vi "drive_setOut.vi"(11 "Drive_Outputs":T1) -> ()   [LabVIEW 2013]
uses:
  drive_outputs.ctl
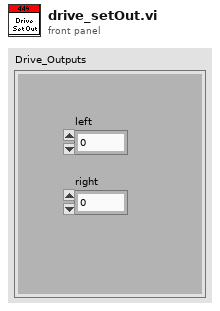
[diagram p1: front panel]
types:
  T1 = typedef "drive_outputs.ctl" = cluster{"left":dbl, "right":dbl}
  T2 = typedef "WPI_MotorControlDeviceRef.ctl" = cluster{"DeviceStatus":errorcluster, "Type":enum16{"PWM", "CAN"}, "PWM":cluster{"Digital Module":T3, "PWM Channel":T4, "DeadBand":T5}, "CAN":cluster{"Device Number":u8, "Control Mode":T6, "Semaphore":T7, "Max Vout":dbl}, "Invert":bool, "TransformRef":T8, "InvTransformRef":T8}
  T3 = typedef "FPGA_TypedefDigitalModule.ctl" = enum16{"Digital Module 1", "Digital Module 2"}
  T4 = typedef "FPGA_DIOPWMChannel.ctl" = enum8{"PWM 1", "PWM 2", "PWM 3", "PWM 4", "PWM 5", "PWM 6", "PWM 7", "PWM 8", "PWM 9", "PWM 10", "Invalid"}
  T5 = typedef "WPI_PWMDeadband.ctl" = cluster{"Name":string, "maxPositivePwm":i32, "minPositivePwm":i32, "centerPwm":i32, "maxNegativePwm":i32, "minNegativePwm":i32, "angularRange":u16}
  T6 = typedef "WPI_CANJaguar_ControlMode.ctl" = enum8{"Percent VBus", "Current", "Speed", "Position", "Voltage"}
  T7 = typedef "Semaphore RefNum" = refnum<k1>
  T8 = typedef "WPI_PWMTransform_ConPane.ctl" = refnum<vi>
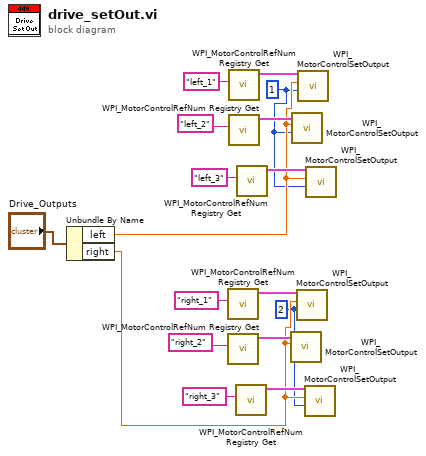
[diagram p0: block diagram]
diagram:
  w1 = u8 2 ("Sync Group")
  w2 = u8 1 ("Sync Group")
  n1 = Unbundle By Name("Drive_Outputs") -> ("left"=w10:dbl, "right"=w3:dbl)
  n2 = call <vilib>:"WPI_MotorControlRefNum Registry Get.vi"("refnum name"="right_1") -> ("MotorControlDevRef"=w9:T2)  [unwired: 9 in, 1 out]
  n3 = call <vilib>:"WPI_MotorControlRefNum Registry Get.vi"("refnum name"="right_2") -> ("MotorControlDevRef"=w7:T2)  [unwired: 9 in, 1 out]
  n4 = call <vilib>:"WPI_MotorControlRefNum Registry Get.vi"("refnum name"="left_1") -> ("MotorControlDevRef"=w16:T2)  [unwired: 9 in, 1 out]
  n5 = call <vilib>:"WPI_MotorControlRefNum Registry Get.vi"("refnum name"="left_2") -> ("MotorControlDevRef"=w14:T2)  [unwired: 9 in, 1 out]
  n6 = call <vilib>:"WPI_MotorControlRefNum Registry Get.vi"("refnum name"="right_3") -> ("MotorControlDevRef"=w5:T2)  [unwired: 9 in, 1 out]
  n7 = call <vilib>:"WPI_MotorControlRefNum Registry Get.vi"("refnum name"="left_3") -> ("MotorControlDevRef"=w12:T2)  [unwired: 9 in, 1 out]
  n8 = call <vilib>:"WPI_MotorControlSetOutput.vi"("Sync Group"=w1, "Output"=w3, "MotorControlDevRef"=w7) -> ()  [unwired: 6 in, 3 out]
  n9 = call <vilib>:"WPI_MotorControlSetOutput.vi"("Sync Group"=w2, "Output"=w10, "MotorControlDevRef"=w14) -> ()  [unwired: 6 in, 3 out]
  n10 = call <vilib>:"WPI_MotorControlSetOutput.vi"("Sync Group"=w1, "Output"=w3, "MotorControlDevRef"=w9) -> ()  [unwired: 6 in, 3 out]
  n11 = call <vilib>:"WPI_MotorControlSetOutput.vi"("Sync Group"=w2, "Output"=w10, "MotorControlDevRef"=w16) -> ()  [unwired: 6 in, 3 out]
  n12 = call <vilib>:"WPI_MotorControlSetOutput.vi"("Sync Group"=w1, "Output"=w3, "MotorControlDevRef"=w5) -> ()  [unwired: 6 in, 3 out]
  n13 = call <vilib>:"WPI_MotorControlSetOutput.vi"("Sync Group"=w2, "Output"=w10, "MotorControlDevRef"=w12) -> ()  [unwired: 6 in, 3 out]
